vi "MFCselection.vi"(5 "MFCsIn":T1[](array[typedef]) {"mDot" format="%_4g"; "Setpoint" format="%.2g"; "MFCcapability"."MaxMdot" format="%_4g"; "MFCcapability"."MinMdot" format="%_4g"}, 6 "MdotMin":dbl=nan, 7 "MdotMax":dbl=nan, 8 "idealSPFraction":dbl=0.7 format="%#_13g", 9 "Mdot":dbl) -> (0 "OffIdeal":dbl, 1 "errorReport":string, 2 "nMFCs":i32, 4 "MFCsOut":T1[](array[typedef]) {"mDot" format="%_4g"; "Setpoint" format="%.2g"; "MFCcapability"."MaxMdot" format="%_4g"; "MFCcapability"."MinMdot" format="%_4g"})   [LabVIEW 2018]
uses:
  MFCdescription.ctl
  MFCcapability.ctl
  ComboRange.ctl
  MFCselectionData.ctl
  SelectionStages.ctl
panel:
  in  "Tab Control":enum32{"I/O", "Page 2", "PrivateData"}(tab)
  in  "UseCurrentMFCs":bool
  out "SuggestedRange":T3
  in  "MeritMeasure":enum16{"MinMFCs", "ClosestToIdeal", "Weighted"}(ring)=enum."ClosestToIdeal"
  out "Array":T4[](array[typedef])
  out "Loops":i32
  out "PrivateData":T5 {"suggestedCombo"."mDot" format="%_4g"; "suggestedCombo"."Setpoint" format="%.2g"; "suggestedCombo"."MFCcapability"."MaxMdot" format="%_4g"; "suggestedCombo"."MFCcapability"."MinMdot" format="%_4g"; "Combos"."mDot" format="%_4g"; "Combos"."Setpoint" format="%.2g"; "Combos"."MFCcapability"."MaxMdot" format="%_4g"; "Combos"."MFCcapability"."MinMdot" format="%_4g"; "MFCs"."mDot" format="%_4g"; "MFCs"."Setpoint" format="%.2g"; "MFCs"."MFCcapability"."MaxMdot" format="%_4g"; "MFCs"."MFCcapability"."MinMdot" format="%_4g"}
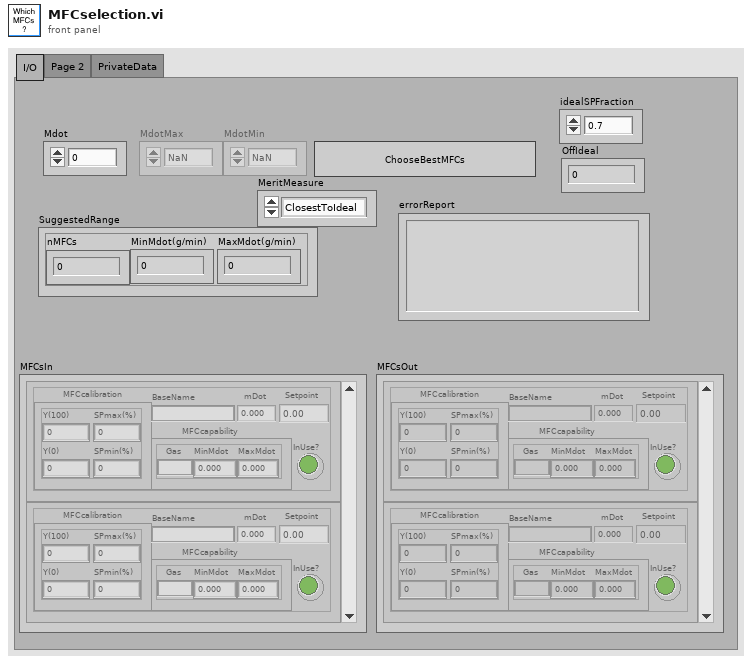
[diagram p1: front panel]
types:
  T1 = typedef "MFCdescription.ctl" = cluster{"BaseName":string, "MFCcalibration":cluster{"Y(100)":dbl, "Y(0)":dbl, "SPmin(%)":dbl, "SPmax(%)":dbl}, "MFCcapability":T2, "InUse?":bool, "Setpoint":dbl, "mDot":dbl}
  T2 = typedef "MFCcapability.ctl" = cluster{"Gas":string, "MinMdot":dbl, "MaxMdot":dbl}
  T3 = typedef "ComboRange.ctl" = cluster{"nMFCs":i32, "MinMdot(g/min)":dbl, "MaxMdot(g/min)":dbl}
  T4 = typedef "SelectionStages.ctl" = enum16{"Initialise", "HaveLimits?", "CurrentComboRange?", "GetAllCombos", "ExtractViableCombos", "EvaluateViableCombos", "WhatNext?", "FinalOutput"}
  T5 = typedef "MFCselectionData.ctl" = cluster{"MFCs":T1[], "Combos":T1[][], "Ranges":T3[], "MeritArray":dbl[], "SuggestedRange":T3, "suggestedCombo":T1[], "Merit":dbl, "nMFCs":i32, "OffCentreArray":dbl[], "OffCentre":dbl, "OverallMinMdot(g/min)":dbl, "OverallMaxMdot(g/min)":dbl, "messages":string}
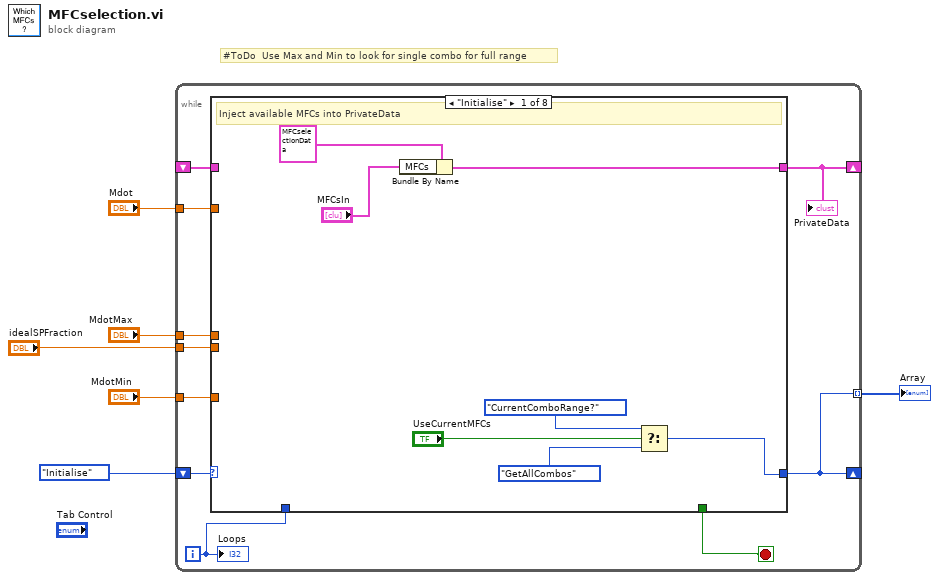
[diagram p0: block diagram]
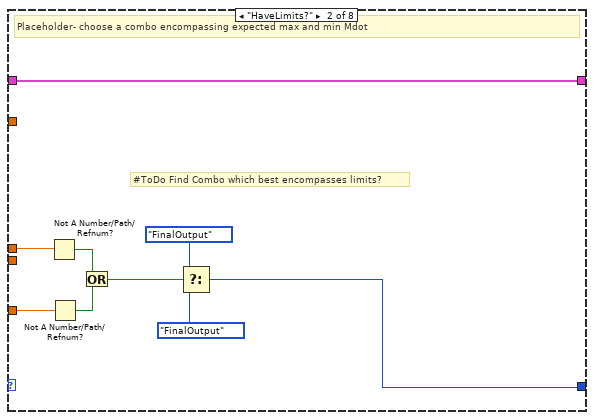
[diagram p2: hidden frame]
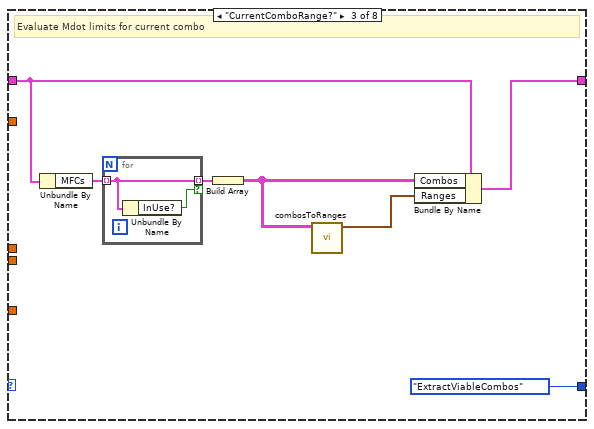
[diagram p3: hidden frame]
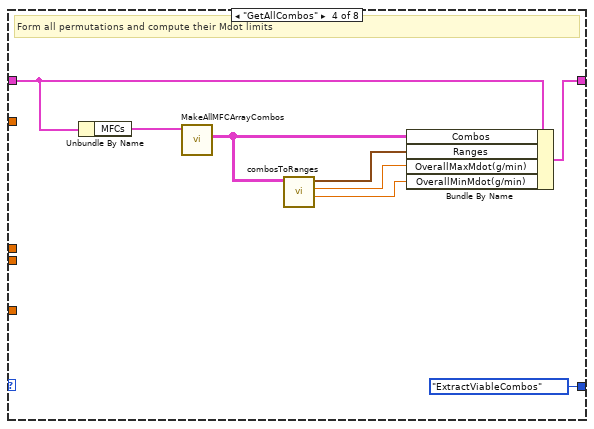
[diagram p4: hidden frame]
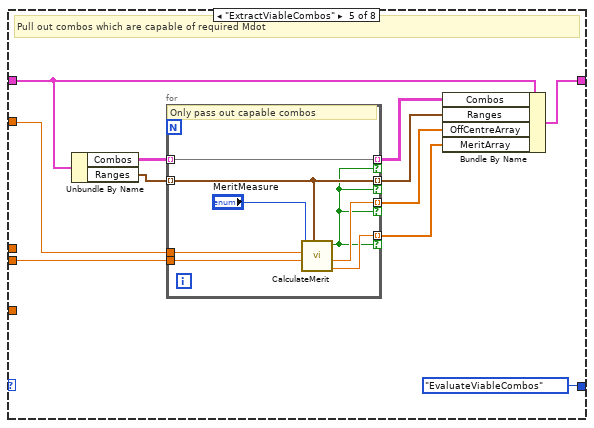
[diagram p5: hidden frame]
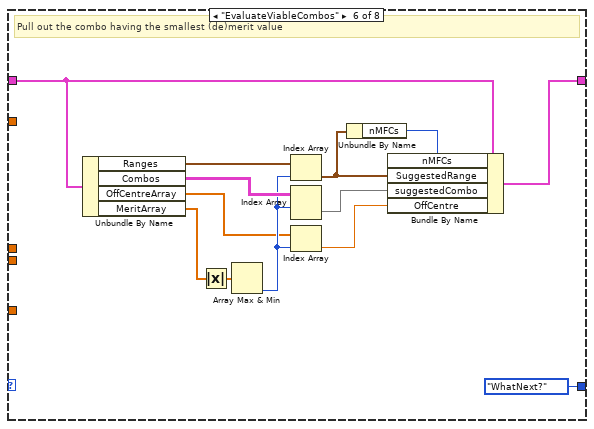
[diagram p6: hidden frame]
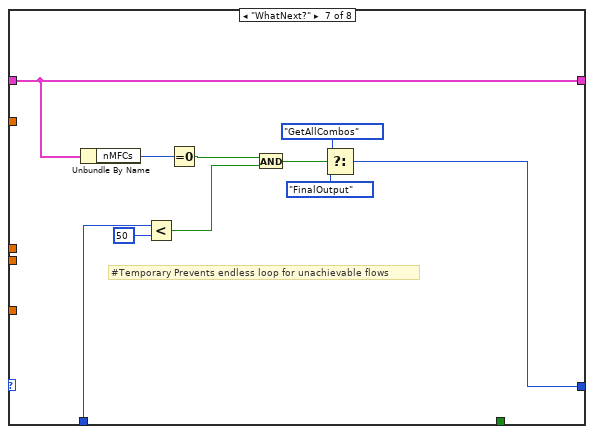
[diagram p7: hidden frame]
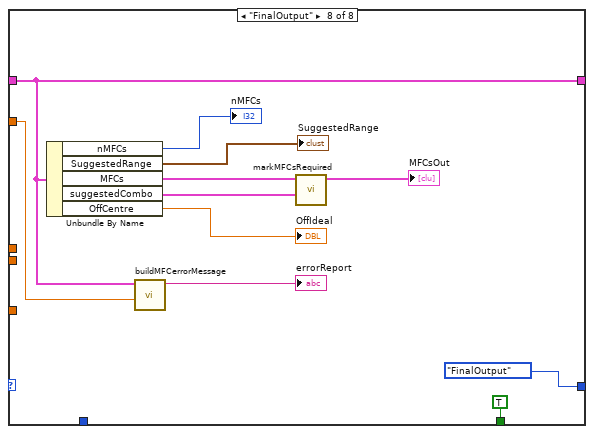
[diagram p8: hidden frame]
diagram:
  # "#ToDo  Use Max and Min to look for single combo for full range"
  n1 = while {
    shift-right: [w8] -> _
    shift-left: SelectionStages."Initialise" -> [w9]
    tunnel: "MdotMax" -> [w16]
    tunnel: "MdotMin" -> [w15]
    tunnel: "Mdot" -> [w14]
    shift-right: [w12] -> _
    shift-left: _ -> [w11]
    tunnel: [w8] -> w2 mode=indexing
    tunnel: "idealSPFraction" -> [w7]
    i -> [w10]
    stop <- w13 stop-if-true
    n2 = case shown="\"Initialise\"" w9 {
      tunnel: w16 -> [_ w32 _ _ _ _ _ _]
      tunnel: w15 -> [_ w31 _ _ _ _ _ _]
      tunnel: [w17 w26 SelectionStages."ExtractViableCombos" SelectionStages."ExtractViableCombos" SelectionStages."EvaluateViableCombos" SelectionStages."WhatNext?" w86 SelectionStages."FinalOutput"] -> w8
      tunnel: w14 -> [_ _ _ _ w59 _ _ w92]
      tunnel: [_ _ _ _ _ _ _ TRUE] -> w13
      tunnel: [w21 w24 w38 w47 w56 w71 w90 w96] -> w12
      tunnel: w11 -> [_ w24 w35 w48 w57 w72 w90 w96]
      tunnel: w10 -> [_ _ _ _ _ _ w85 _]
      tunnel: w7 -> [_ _ _ _ w50 _ _ _]
      frame "Initialise" {
        # "Inject available MFCs into PrivateData"
        n3 = Bundle By Name(cluster=T5 {"MFCs"=[], "Combos"=[], "Ranges"=[], "MeritArray"=[], "SuggestedRange"={"nMFCs"=0, "MinMdot(g/min)"=0.0, "MaxMdot(g/min)"=0.0}, "suggestedCombo"=[], "Merit"=0.0, "nMFCs"=0, "OffCentreArray"=[], "OffCentre"=0.0, "OverallMinMdot(g/min)"=0.0, "OverallMaxMdot(g/min)"=0.0, "messages"=""}, "MFCs"="MFCsIn") -> (w21:T5)
        n4 = Select(t=SelectionStages."CurrentComboRange?", s="UseCurrentMFCs", f=SelectionStages."GetAllCombos") -> (s? t:f=w17:T4)
      }
      frame "HaveLimits?" {
        # "#ToDo Find Combo which best encompasses limits?"
        # "Placeholder- choose a combo encompassing expected max and min Mdot"
        n5 = Not A Number/Path/Refnum?(number/path/refnum=w32) -> (NaN/Path/Refnum?=w30:bool)
        n6 = Not A Number/Path/Refnum?(number/path/refnum=w31) -> (NaN/Path/Refnum?=w29:bool)
        n7 = Or(x=w30, y=w29) -> (x .or. y?=w28:bool)
        n8 = Select(t=SelectionStages."FinalOutput", s=w28, f=SelectionStages."FinalOutput") -> (s? t:f=w26:T4)
      }
      frame "CurrentComboRange?" {
        # "Evaluate Mdot limits for current combo"
        n9 = Unbundle By Name(w35) -> ("MFCs"=w34:T1[])
        n10 = for {
          tunnel: w34 -> [w41] mode=indexing
          tunnel: [w41] -> w33 mode=indexing if=w40
          n11 = Unbundle By Name(w41) -> ("InUse?"=w40:bool)
        }
        n12 = Build Array(w33) -> (w37:T1[][])
        n13 = call "combosToRanges.vi"("combosIn"=w37) -> ("rangesOut"=w39:T3[])  [unwired: 8 in, 2 out]
        n14 = Bundle By Name(cluster=w35, "Combos"=w37, "Ranges"=w39) -> (w38:T5)
      }
      frame "GetAllCombos" {
        # "Form all permutations and compute their Mdot limits"
        n15 = Unbundle By Name(w48) -> ("MFCs"=w49:T1[])
        n16 = call "MakeAllMFCArrayCombos.vi"("EvaluatedMFCs"=w49) -> ("EveryCombination"=w46:T1[][])  [unwired: 10 in]
        n17 = call "combosToRanges.vi"("combosIn"=w46) -> ("OverallMinMdot(g/min)"=w42:dbl, "OverallMaxMdot(g/min)"=w43:dbl, "rangesOut"=w45:T3[])  [unwired: 8 in]
        n18 = Bundle By Name(cluster=w48, "Combos"=w46, "Ranges"=w45, "OverallMaxMdot(g/min)"=w43, "OverallMinMdot(g/min)"=w42) -> (w47:T5)
      }
      frame "ExtractViableCombos" {
        # "Pull out combos which are capable of required Mdot"
        n19 = Unbundle By Name(w57) -> ("Combos"=w58:T1[][], "Ranges"=w60:T3[])
        n20 = for {
          tunnel: w60 -> [w66] mode=indexing
          tunnel: w59 -> [w67]
          tunnel: [w68] -> w55 mode=indexing if=w63
          tunnel: w58 -> [w68] mode=indexing
          tunnel: [w66] -> w54 mode=indexing if=w63
          tunnel: [w65] -> w52 mode=indexing if=w63
          tunnel: [w64] -> w51 mode=indexing if=w63
          tunnel: w50 -> [w61]
          # "Only pass out capable combos"
          n21 = call "CalculateMerit.vi"("RangeInfo"=w66, "idealSPFraction"=w61, "Target"=w67, "MeritMeasure"="MeritMeasure") -> ("Merit (smaller is better)"=w65:dbl, "OffsetFromIdeal"=w64:dbl, "In Range?"=w63:bool)  [unwired: 4 in, 1 out]
        }
        n22 = Bundle By Name(cluster=w57, "Combos"=w55, "Ranges"=w54, "OffCentreArray"=w51, "MeritArray"=w52) -> (w56:T5)
      }
      frame "EvaluateViableCombos" {
        # "Pull out the combo having the smallest (de)merit value"
        n23 = Unbundle By Name(w72) -> ("Ranges"=w80:T3[], "Combos"=w81:T1[][], "OffCentreArray"=w69:dbl[], "MeritArray"=w70:dbl[])
        n24 = Absolute Value(x=w70) -> (abs(x)=w79:dbl[])
        n25 = Array Max & Min(array=w79) -> (min index (indices)=w78:i32)  [unwired: 3 out]
        n26 = Index Array(array=w80, index=w78) -> (element=w75:T3)
        n27 = Index Array(array=w81, index (row)=w78) -> (element=w74:T1[])  [unwired: 1 in]
        n28 = Index Array(array=w69, index=w78) -> (element=w73:dbl)
        n29 = Unbundle By Name(w75) -> ("nMFCs"=w76:i32)
        n30 = Bundle By Name(cluster=w72, "nMFCs"=w76, "SuggestedRange"=w75, "suggestedCombo"=w74, "OffCentre"=w73) -> (w71:T5)
      }
      frame "WhatNext?" {
        # "#Temporary Prevents endless loop for unachievable flows"
        n31 = Unbundle By Name(w90) -> ("nMFCs"=w91:i32)
        n32 = Less?(x=w85, y=50) -> (x < y?=w82:bool)
        n33 = Equal To 0?(x=w91) -> (x = 0?=w89:bool)
        n34 = And(x=w89, y=w82) -> (x .and. y?=w83:bool)
        n35 = Select(t=SelectionStages."GetAllCombos", s=w83, f=SelectionStages."FinalOutput") -> (s? t:f=w86:T4)
      }
      frame "FinalOutput" {
        n36 = Unbundle By Name(w96) -> ("nMFCs"=→"nMFCs":i32, "SuggestedRange"=→"SuggestedRange":T3, "MFCs"=w99:T1[], "suggestedCombo"=w97:T1[], "OffCentre"=→"OffIdeal":dbl)
        n37 = call "buildMFCerrorMessage.vi"("Mdot"=w92, "data"=w96) -> ("finalMessage"=→"errorReport":string)  [unwired: 9 in]
        n38 = call "markMFCsRequired.vi"("suggestedCombo"=w97, "MFCsIn"=w99) -> ("MFCsOut"=→"MFCsOut":T1[])  [unwired: 9 in]
      }
    }
    "PrivateData" <- w12
    "Loops" <- w10
  }
  "Array" <- w2
